vi "set_params.vi"(8 "error in (no error)":errorcluster caption="entrée d'erreur (pas d'erreur)", 11 "MiniBatchKMeans.lvclass 2":refnum<class "MiniBatchKMeans.lvclass">) -> (0 "error out":errorcluster caption="sortie d'erreur", 3 "MiniBatchKMeans.lvclass":refnum<class "MiniBatchKMeans.lvclass">)   [LabVIEW 2020, in "MiniBatchKMeans.lvclass"]
uses:
  MiniBatchKMeans.lvclass
  MiniBatchKMeans.lvclass/MiniBatchKMeans.ctl
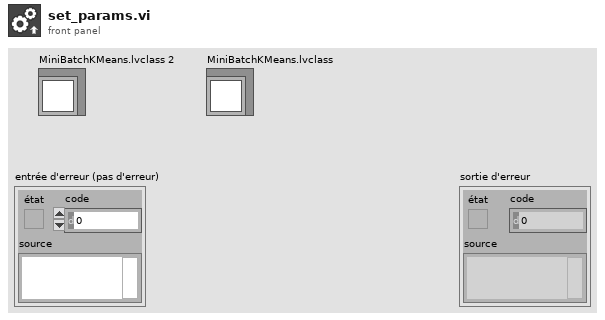
[diagram p1: front panel]
types:
  T1 = typedef "mini_batch_kmeans_params.ctl" = cluster{"n_clusters":dbl, "init":cluster{"init_type":string, "init_list":dbl[][]}, "max_iter":dbl, "batch_size":dbl, "verbose":dbl, "compute_labels":bool, "random_state":dbl, "tol":dbl, "max_no_improvement":dbl, "init_size":cluster{"init_size_type":string, "init_size_int":dbl}, "n_init":dbl, "reassignment_ratio":dbl}
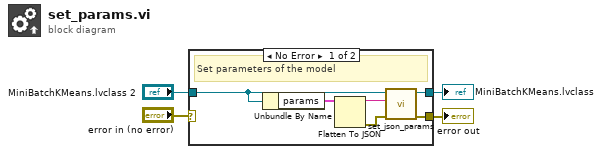
[diagram p0: block diagram]
diagram:
  n1 = case shown="No Error" "error in (no error)" {
    selector: "error in (no error)" -> [_ w12]
    tunnel: [w7 w12] -> w3
    tunnel: [w8 w11] -> w1
    tunnel: "MiniBatchKMeans.lvclass 2" -> [w5 w11]
    frame No Error {
      # "Set parameters of the model"
      n2 = Unbundle By Name(w5) -> ("params"=w10:T1)
      n3 = Flatten To JSON(anything=w10) -> (JSON string=w9:string, 11:w6:errorcluster)  [unwired: 2 in]
      n4 = call-dynamic "set_json_params.vi"("error in (no error)"=w6, "params"=w9, "Model en entrée"=w5) -> ("error out"=w7:errorcluster, "Model en sortie"=w8:refnum<class "MiniBatchKMeans.lvclass">)  [unwired: 7 in]
    }
    frame Error {
    }
  }
  "error out" <- w3
  "MiniBatchKMeans.lvclass" <- w1
